vi "RSZVB Set Calibration Power Generator Offset.vi"(6 "Generator Number (1)":i32=1, 7 "Cal Power Generator Offset (0)":dbl format="%^.3e", 8 "error in (no error)":errorcluster {"code" format="%.0x"}, 9 "Port Number (1)":i32=1, 10 "Channel (1)":i32=1, 11 "VISA session":refnum<visa-resource-name>) -> (0 "error out":errorcluster {"code" format="%.0x"}, 3 "dup VISA session":refnum<visa-resource-name>)   [LabVIEW 2011]
doc: "This VI specifies a gain (positive values) or an attenuation (negative values) in the signal path between the external generator and the calibrated reference plane. The value has no impact on the generator power. \n\nNote(s):\n\n(1) This VI is availble only with R&S ZVA and ZVT instruments. \n\nRemote-control command(s):\nSOURce<Ch>:POWer<Pt>:CORRection:GENerator<Gen>:LEVel:OFFSet <offset>"
uses:
  _utility/RSZVB Global Data.vi
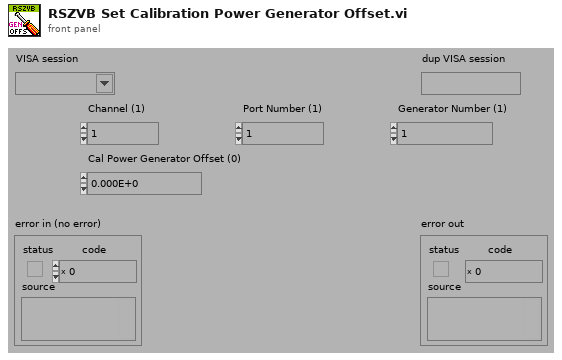
[diagram p1: front panel]
types:
  T1 = cluster{"Error Checking (T: On)":bool, "Installed Options":string[], "Data Valid?":bool, "Ports":i32, "Model":string[], "Option Checking (T: On)":bool}[]
  T2 = cluster{"Error Checking (T: On)":bool, "Installed Options":string[], "Data Valid?":bool, "Ports":i32, "Model":string[], "Option Checking (T: On)":bool}
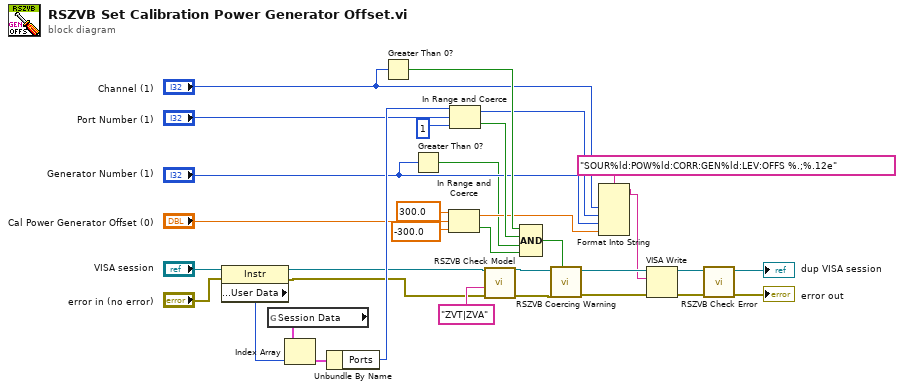
[diagram p0: block diagram]
diagram:
  n1 = property class="Instr"(reference="VISA session", error in="error in (no error)") -> (reference out=w2:refnum<visa-resource-name>, error out=w1:errorcluster, "General Settings:User Data"=w21:u32)
  n2 = global read "RSZVB Global Data.vi" "Session Data"() -> (w22:T1)
  n3 = Index Array(array=w22, index=w21) -> (element=w23:T2)
  n4 = Unbundle By Name(w23) -> ("Ports"=w19:i32)
  n5 = Greater Than 0?(x="Channel (1)") -> (x > 0?=w25:bool)
  n6 = Greater Than 0?(x="Generator Number (1)") -> (x > 0?=w7:bool)
  n7 = In Range and Coerce(upper limit=300.0, x="Cal Power Generator Offset (0)", lower limit=-300.0) -> (coerced(x)=w10:dbl, In Range?=w8:bool)
  n8 = In Range and Coerce(upper limit=w19, x="Port Number (1)", lower limit=1) -> (coerced(x)=w18:i32, In Range?=w17:bool)
  n9 = call "RSZVB Check Model.vi"("error in (no error)"=w1, "Model"="ZVT|ZVA" ("Options"), "VISA session"=w2) -> ("error out"=w4:errorcluster, "dup VISA session"=w3:refnum<visa-resource-name>)  [unwired: 7 in]
  n10 = Compound Arithmetic op=AND(w25, w17, w7, w8) -> (w24:bool)
  n11 = call "RSZVB Coercing Warning.vi"("In Range?"=w24, "error in (no error)"=w4, "VISA session"=w3) -> ("error out"=w32:errorcluster, "dup VISA session"=w33:refnum<visa-resource-name>)  [unwired: 7 in]
  n12 = Format Into String(format string="SOUR%ld:POW%ld:CORR:GEN%ld:LEV:OFFS %.;%.12e", "Channel (1)", w18, "Generator Number (1)", w10) -> (resulting string=w28:string)  [unwired: 2 in, 1 out]
  n13 = VISA Write(VISA resource name=w33, write buffer=w28, error in (no error)=w32) -> (VISA resource name out=w30:refnum<visa-resource-name>, error out=w31:errorcluster)  [unwired: 1 out]
  n14 = call "RSZVB Check Error.vi"("error in (no error)"=w31, "VISA session"=w30) -> ("error out"=→"error out":errorcluster, "dup VISA session"=→"dup VISA session":refnum<visa-resource-name>)  [unwired: 8 in]
